vi "Read Next Message_sushu.vi"(0 "Queue In":cluster{"Q":T1, "Name":string}, 1 "ignore error on termination message (F)":bool, 5 "termination list ([Exit])":string[](array[string])=["Exit"], 7 "timeout (1 ms)":i32=1, 11 "error in":errorcluster) -> (2 "Previous State + Arguments":string, 3 "exit process?":bool, 4 "Queue Out":cluster{"Q":T1, "Name":string}, 6 "Current State":string, 8 "Arguments":string, 10 "message value":string, 12 "acknowledge":bool, 13 "timed out?":bool, 14 "message":T2, 15 "error out":errorcluster)   [LabVIEW 2021]
doc: "基于AMC二次封装的读取队列元素的模块。\n20140304\nReturns the next message from the message queue passed in. If the returned message matches any of the message names listed in \"termination list\" the \"exit process?\" indicator will return True."
uses:
  <vilib>/NI/AMC/Message.ctl
  <vilib>/NI/Tools/Keyed Array/KeyedArray.ctl
  <vilib>/NI/AMC/Message Queue.ctl
  <vilib>/NI/AMC/Read Termination Message.vi
  <vilib>/NI/AMC/Create Single Message.vi
  <vilib>/NI/AMC/Globals.vi
  <vilib>/NI/AMC/AMC.lvlib
  <vilib>/NI/Tools/Keyed Array/Tools_KeyedArray.lvlib
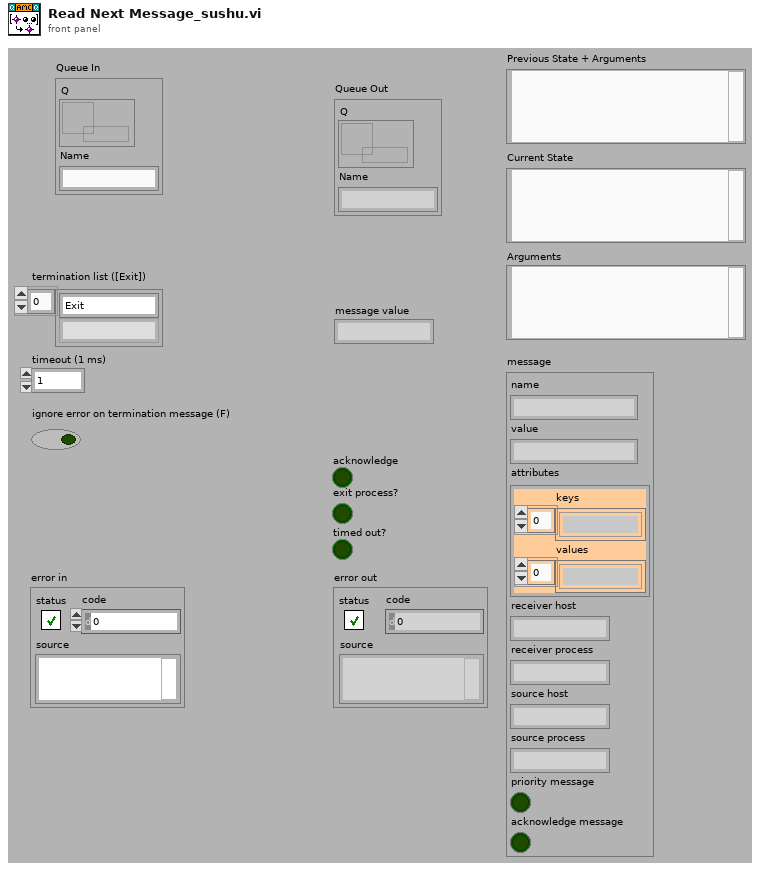
[diagram p1: front panel]
types:
  T1 = typedef "AMC.lvlib/Message Queue.ctl" = refnum<queue>
  T2 = typedef "AMC.lvlib/Message.ctl" = cluster{"name":string, "value":string, "attributes":T3, "receiver host":string, "receiver process":string, "source host":string, "source process":string, "priority message":bool, "acknowledge message":bool}
  T3 = typedef "Tools_KeyedArray.lvlib/KeyedArray.ctl" = cluster{"keys":string[], "values":string[]}
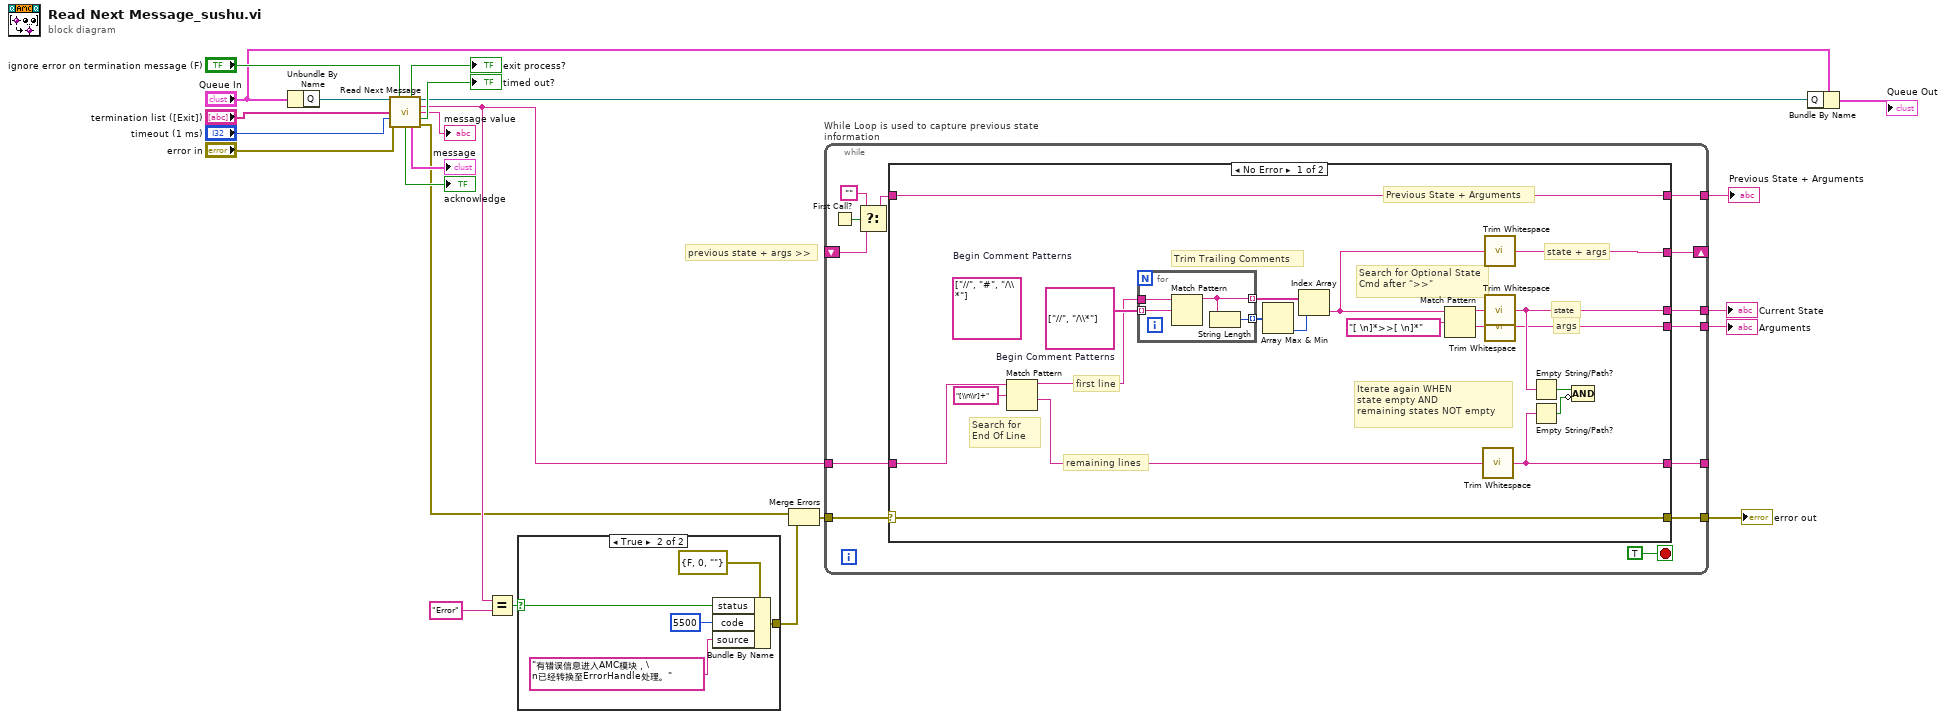
[diagram p0: block diagram]
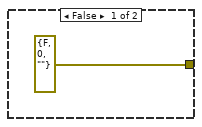
[diagram p2: hidden frame]
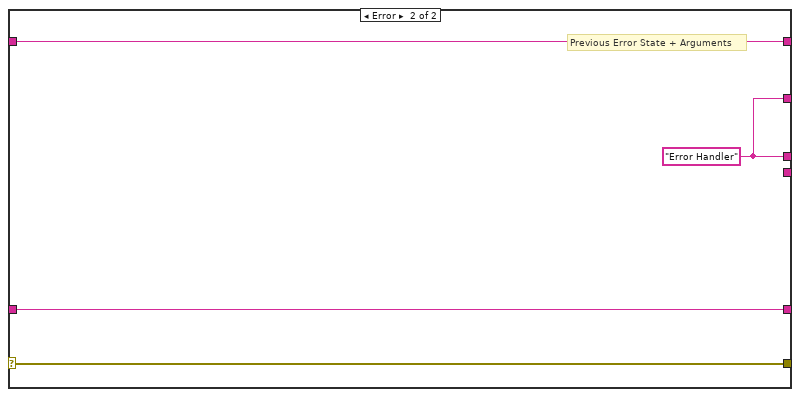
[diagram p3: hidden frame]
diagram:
  # "previous state + args >>"
  n1 = Unbundle By Name("Queue In") -> ("Q"=w14:T1)
  n2 = call <vilib>:"Read Next Message.vi"("message queue in"=w14, "ignore error on termination message (F)"="ignore error on termination message (F)", "termination list ([Exit])"="termination list ([Exit])", "timeout (1 ms)"="timeout (1 ms)", "error in"="error in") -> ("exit process?"=→"exit process?":bool, "message queue out"=w13:T1, "message name"=w6:string, "message value"=→"message value":string, "timed out?"=→"timed out?":bool, "acknowledge"=→"acknowledge":bool, "message"=→"message":T2, "error out"=w3:errorcluster)  [unwired: 3 in]
  n3 = Equal?(x=w6, y="Error") -> (x = y?=w2:bool)
  n4 = case shown="True" w2 {
    selector: w2 -> [_ w26]
    tunnel: [errorcluster {"status"=FALSE, "code"=0, "source"=""} ("error constant") w25] -> w1
    frame False {
    }
    frame True {
      n5 = Bundle By Name(cluster=errorcluster {"status"=FALSE, "code"=0, "source"=""} ("error constant"), "status"=w26, "code"=5500, "source"="有错误信息进入AMC模块，\n已经转换至ErrorHandle处理。") -> (w25:errorcluster)
    }
  }
  n6 = Merge Errors(w3, w1) -> (w4:errorcluster)
  n7 = while "While Loop is used to capture previous state information" {
    tunnel: [w42] -> _
    tunnel: w6 -> [w41]
    tunnel: w4 -> [w40]
    tunnel: [w39] -> w10
    tunnel: [w38] -> w9
    shift-right: [w36] -> _
    shift-left: _ -> [w34]
    tunnel: [w31] -> w8
    tunnel: [w30] -> w7
    stop <- TRUE stop-if-true
    n8 = First Call?() -> (First Call?: T/F=w35:bool)
    n9 = Select(t="", s=w35, f=w34) -> (s? t:f=w33:string)
    n10 = case shown="No Error" w40 {
      selector: w40 -> [w56 w67]
      tunnel: [w59 w70] -> w42
      tunnel: [w62 w68] -> w39
      tunnel: [w61 _] -> w38
      tunnel: w41 -> [w60 w70]
      tunnel: [w58 w68] -> w36
      tunnel: w33 -> [w57 w69]
      tunnel: [w57 w69] -> w31
      tunnel: [w56 w67] -> w30
      frame No Error {
        (unwired) string[] ["//", "#", "/\\*"]  # Begin Comment Patterns
        w54 = string[] ["//", "/\\*"]  # Begin Comment Patterns
        # "state + args"
        # "remaining lines"
        # "first line"
        # "Search for End Of Line"
        # "Iterate again WHEN\nstate empty AND\nremaining states NOT empty"
        # "args"
        # "state"
        # "Search for Optional State Cmd after \">>\""
        # "Trim Trailing Comments"
        # "Previous State + Arguments"
        n11 = Match Pattern(string=w60, regular expression="[\\n\\r]+") -> (before substring=w44:string, after substring=w55:string)  [unwired: 1 in, 2 out]
        n12 = for {
          tunnel: w44 -> [w66]
          tunnel: [w64] -> w51 mode=indexing
          tunnel: w54 -> [w65] mode=indexing
          tunnel: [w63] -> w53 mode=indexing
          n13 = Match Pattern(string=w66, regular expression=w65) -> (before substring=w64:string)  [unwired: 1 in, 3 out]
          n14 = String Length(string=w64) -> (length=w63:i32)
        }
        n15 = Array Max & Min(array=w53) -> (min index (indices)=w52:i32)  [unwired: 3 out]
        n16 = Index Array(array=w51, index=w52) -> (element=w43:string)
        n17 = Match Pattern(string=w43, regular expression="[ \n]*>>[ \n]*") -> (before substring=w49:string, after substring=w48:string)  [unwired: 1 in, 2 out]
        n18 = call <vilib>:"Trim Whitespace.vi"("string"=w55) -> ("trimmed string"=w59:string)  [unwired: 1 in]
        n19 = call <vilib>:"Trim Whitespace.vi"("string"=w43) -> ("trimmed string"=w58:string)  [unwired: 1 in]
        n20 = call <vilib>:"Trim Whitespace.vi"("string"=w49) -> ("trimmed string"=w62:string)  [unwired: 1 in]
        n21 = call <vilib>:"Trim Whitespace.vi"("string"=w48) -> ("trimmed string"=w61:string)  [unwired: 1 in]
        n22 = Empty String/Path?(string/path=w62) -> (empty?=w47:bool)
        n23 = Empty String/Path?(string/path=w59) -> (empty?=w46:bool)
        n24 = Compound Arithmetic op=AND(w47, invert w46) -> ()  [unwired: 1 out]
      }
      frame Error {
        w68 = "Error Handler"
        # "Previous Error State + Arguments"
      }
    }
  }
  "error out" <- w7
  "Arguments" <- w9
  "Current State" <- w10
  "Previous State + Arguments" <- w8
  n25 = Bundle By Name(cluster="Queue In", "Q"=w13) -> (→"Queue Out":cluster{"Q":T1, "Name":string})
